vi "Create Request.vi"(6 "wait for reply (T)":bool=TRUE, 8 "error in (no error)":errorcluster, 9 "Create":bool, 10 "Simple Reason String":string) -> (0 "error out":errorcluster, 1 "timed out?":bool, 2 "Reply Payload":T1)   [LabVIEW 2024, in "DQMH Power Requests.lvlib"]
doc: "Creates or destroys Power Request. Requires Simple Reason String to create request. Returns true is successful.\n_____\nCreated using Delacor QMH Event Scripter 4.2.1.88.\n\n<b>Note:</b> This VI was modified by the <b>Validate DQMH Module</b> tool to return an error if the reply times out.\n\n<b>Note:</b> This VI was modified by the <b>Validate DQMH Module</b> tool to turn off automatic error handling."
uses:
  DQMH Power Requests.lvlib
  Create Request (Reply Payload)--cluster.ctl
  Create Request Argument--cluster.ctl
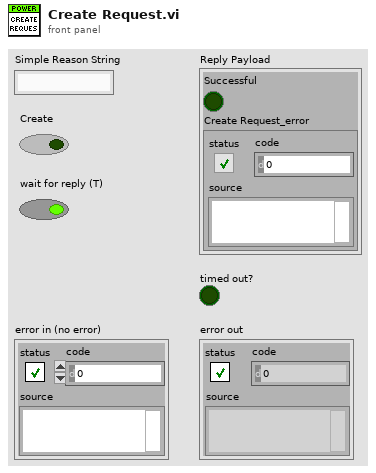
[diagram p1: front panel]
types:
  T1 = typedef "DQMH Power Requests.lvlib/Create Request (Reply Payload)--cluster.ctl" = cluster{"Successful":bool, "Create Request_error":errorcluster}
  T2 = typedef "DQMH Power Requests.lvlib/Create Request Argument--cluster.ctl" = cluster{"Simple Reason String":string, "Create":bool, "Wait Notifier":refnum<notifier>, "wait for reply":bool}
  T3 = typedef "DQMH Power Requests.lvlib/Request Events--cluster.ctl" = cluster{"Stop Module":refnum<user-event>, "Show Panel":refnum<user-event>, "Hide Panel":refnum<user-event>, "Get Module Execution Status":refnum<user-event>, "Show Diagram":refnum<user-event>, "Create Request":refnum<user-event>, "System Required":refnum<user-event>, "Display Required":refnum<user-event>}
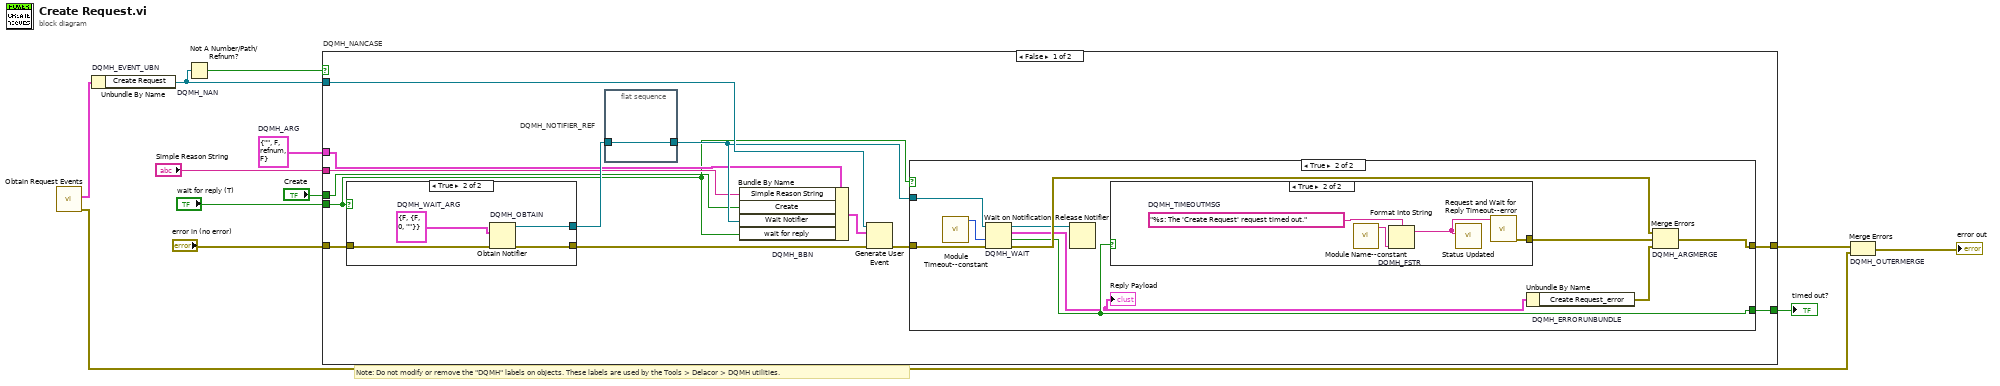
[diagram p0: block diagram]
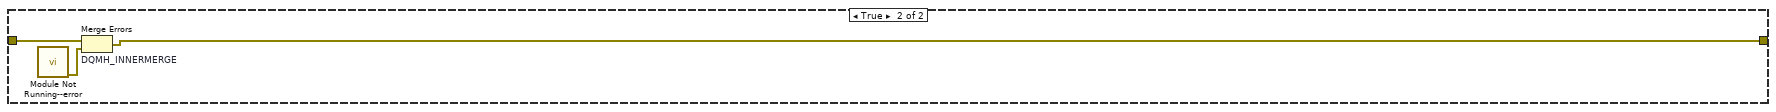
[diagram p5: hidden frame]
diagram:
  w6 = T2 {"Simple Reason String"="", "Create"=FALSE, "Wait Notifier"=refnum, "wait for reply"=FALSE}  # DQMH_ARG
  # "Note: Do not modify or remove the \"DQMH\" labels on objects. These labels are used by the Tools > Delacor > DQMH utilities."
  n1 = call "Obtain Request Events.vi"() -> ("error out"=w2:errorcluster, "DQMH Power Requests Request Events"=w1:T3)  [unwired: 10 in]
  n2 = Unbundle By Name "DQMH_EVENT_UBN"(w1) -> ("Create Request"=w10:refnum<user-event>)
  n3 = Not A Number/Path/Refnum? "DQMH_NAN"(number/path/refnum=w10) -> (NaN/Path/Refnum?=w9:bool)
  n4 = case "DQMH_NANCASE" shown="False" w9 {
    tunnel: "error in (no error)" -> [w25 w49]
    tunnel: w10 -> [w23 _]
    tunnel: [w20 w48] -> w7
    tunnel: [w21 _] -> w8
    tunnel: w6 -> [w16 _]
    tunnel: "Simple Reason String" -> [w15 _]
    tunnel: "Create" -> [w14 _]
    tunnel: "wait for reply (T)" -> [w13 _]
    frame False {
      n5 = case shown="True" w13 {
        tunnel: w25 -> [w42 w46]
        tunnel: [w42 w45] -> w22
        tunnel: [_ w43] -> w18
        frame False {
        }
        frame True {
          w44 = T1 {"Successful"=FALSE, "Create Request_error"={"status"=FALSE, "code"=0, "source"=""}}  # DQMH_WAIT_ARG
          n6 = Obtain Notifier "DQMH_OBTAIN"(notification data type=w44, error in (no error)=w46) -> (notifier out=w43:refnum<notifier>, error out=w45:errorcluster)  [unwired: 2 in, 1 out]
        }
      }
      n7 = flat-sequence "DQMH_NOTIFIER_REF" {
        tunnel: w18 -> [w26]
        tunnel: [w26] -> w17
        frame #0 {
        }
      }
      n8 = Bundle By Name "DQMH_BBN"(cluster=w16, "Simple Reason String"=w15, "Create"=w14, "Wait Notifier"=w17, "wait for reply"=w13) -> (w19:T2)
      n9 = Generate User Event(user event=w23, event data cluster=w19, error in=w22) -> (error out=w24:errorcluster)  [unwired: 1 in, 1 out]
      n10 = case shown="True" w13 {
        tunnel: w24 -> [w27 w37]
        tunnel: w17 -> [_ w35]
        tunnel: [_ w33] -> w21
        tunnel: [w27 w32] -> w20
        frame False {
        }
        frame True {
          n11 = call "Module Timeout--constant.vi"() -> ("Module Timeout"=w29:i32)  [unwired: 11 in]
          n12 = Wait on Notification "DQMH_WAIT"(notifier=w35, timeout in ms (-1)=w29, error in (no error)=w37) -> (notifier out=w34:refnum<notifier>, notification=w30:T1, timed out?=w33:bool, error out=w36:errorcluster)  [unwired: 1 in]
          "Reply Payload" <- w30
          n13 = Release Notifier(notifier=w34) -> ()  [unwired: 2 in, 3 out]
          n14 = case shown="True" w33 {
            tunnel: [_ w38] -> w28
            frame False {
            }
            frame True {
              w41 = "%s: The 'Create Request' request timed out."  # DQMH_TIMEOUTMSG
              n15 = call "Module Name--constant.vi"() -> ("Module Name"=w40:string)  [unwired: 11 in]
              n16 = Format Into String "DQMH_FSTR"(format string=w41, w40) -> (resulting string=w39:string)  [unwired: 2 in, 1 out]
              n17 = call "Status Updated.vi"("Status"=w39) -> ()  [unwired: 10 in, 1 out]
              n18 = call "Request and Wait for Reply Timeout--error.vi"("Error Message"=w39) -> ("error out"=w38:errorcluster)  [unwired: 10 in]
            }
          }
          n19 = Unbundle By Name "DQMH_ERRORUNBUNDLE"(w30) -> ("Create Request_error"=w31:errorcluster)
          n20 = Merge Errors "DQMH_ARGMERGE"(w36, w28, w31) -> (w32:errorcluster)
        }
      }
    }
    frame True {
      n21 = call "Module Not Running--error.vi"() -> ("error out"=w47:errorcluster)  [unwired: 11 in]
      n22 = Merge Errors "DQMH_INNERMERGE"(w49, w47) -> (w48:errorcluster)
    }
  }
  "timed out?" <- w8
  n23 = Merge Errors "DQMH_OUTERMERGE"(w7, w2) -> (→"error out":errorcluster)
